vi "SQLiteConfig.vi"(4 "ConfigCommand":T2, 5 "error in (no error)":errorcluster, 7 "KeyDataIn":string, 8 "Parameter":T1) -> (0 "error out":errorcluster, 1 "All Data":string[][](array[string]), 2 "KeyData":string, 3 "AvailableVersions":string[](array[string]))   [LabVIEW 2023]
doc: "*-----------------------------------------------------\n* Author: SWatts\n*\n* VI Description: Configuration dialog\n* \n*\n* Error handling: All errors passed out\n*\n* Pre-condition: \n*\n* Post-condition: None\n*\n* Revision History:\n*\n* Rev Date Author Description \n* 01 30/04/2014 SWatts First issue\n*\n*-----------------------------------------------------"
uses:
  Datamanager.ctl
  Controls/SystemConfigData.ctl
  Database/SystemdBCommands.ctl
  System Config Data Manager Parameter.ctl
  ConfigCommand.ctl
panel:
  out "KeyNames":string[](array[string])
  # "Local"
  # "Output"
  # "Input"
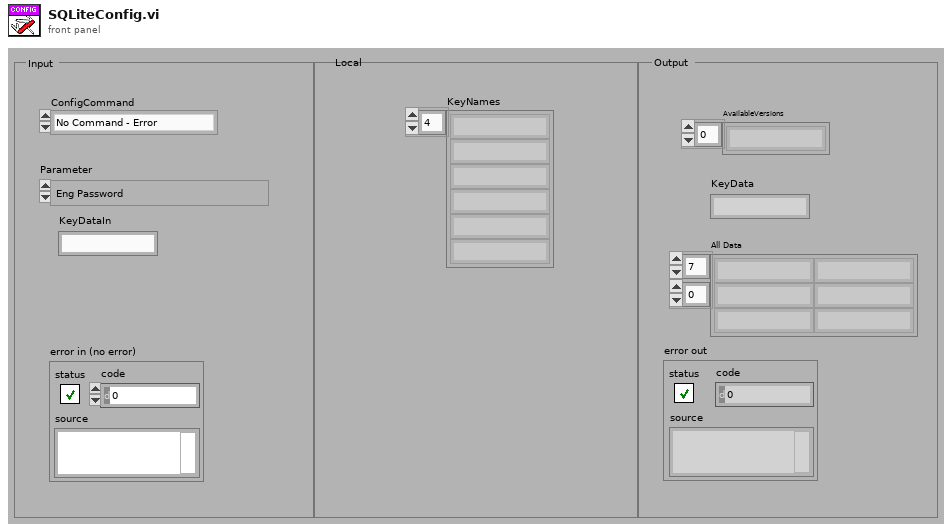
[diagram p1: front panel]
types:
  T1 = typedef "System Config Data Manager Parameter.ctl" = enum16{"Eng Password", "DSN Connection", "User Password", "RunStatus", "InitialDataPath", "helpFilePath", "ErrorFilepath", "DatalogPath", "Hello"}
  T2 = typedef "ConfigCommand.ctl" = enum16{"No Command - Error", "Initialise Config SQLite", "Save Config", "Get Key", "Set Key", "Update Key", "Get Latest Config Data", "Get Config Data for Version", "Get Default Config Data"}
  T3 = typedef "Datamanager.ctl" = enum16{"System Config"}
  T4 = typedef "SystemConfigData.ctl" = cluster{"KeyNames":string[], "Section":string, "Version":string, "KeyData":string[]}
  T5 = typedef "SystemdBCommands.ctl" = enum16{"No Command - Error", "Set Filepath", "Connect dB", "Disconnect dB", "Start Transaction", "Commit", "Rollback", "Describe Table", "Select All From Table", "Fetch Query", "Count Records In Table", "Get User Information", "Get System Config", "Insert New System Config", "UPDATE User Info", "Insert New User", "Get Versions", "Update Key", "Set Version to Default", "Get Default Version", "INSERT Error", "UPDATE Error", "DELETE Errors", "Get All Errors", "Get #Errors for Error"}
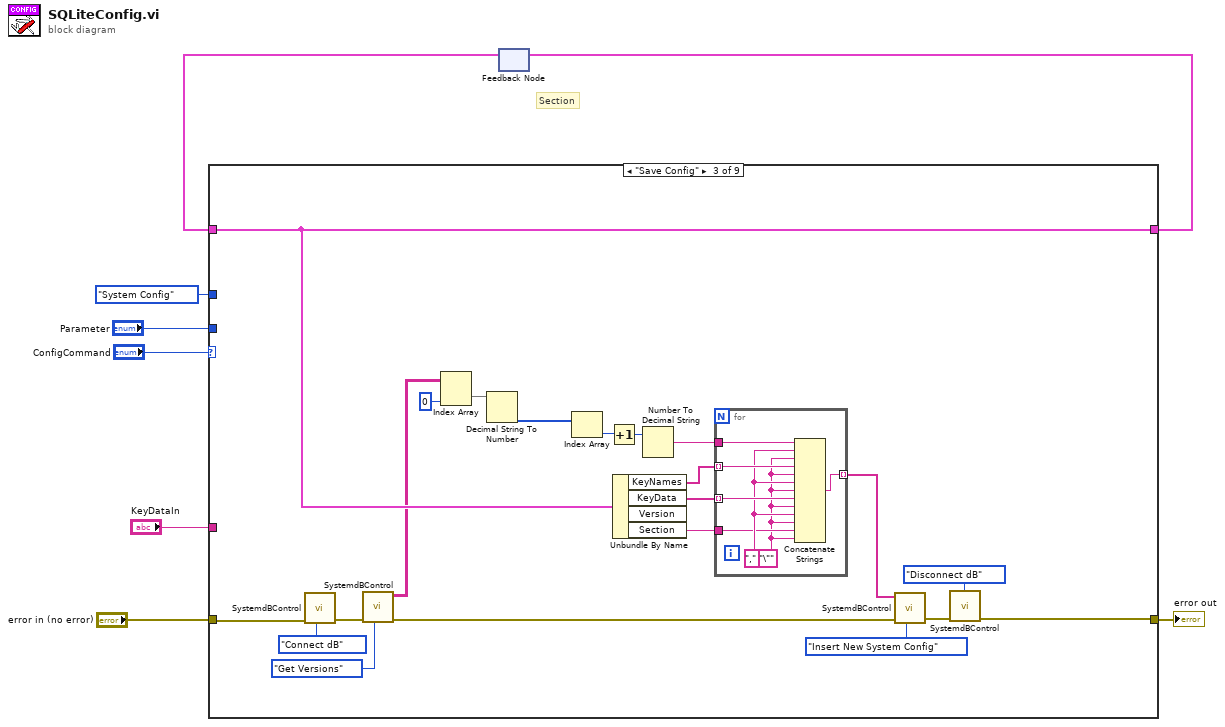
[diagram p0: block diagram]
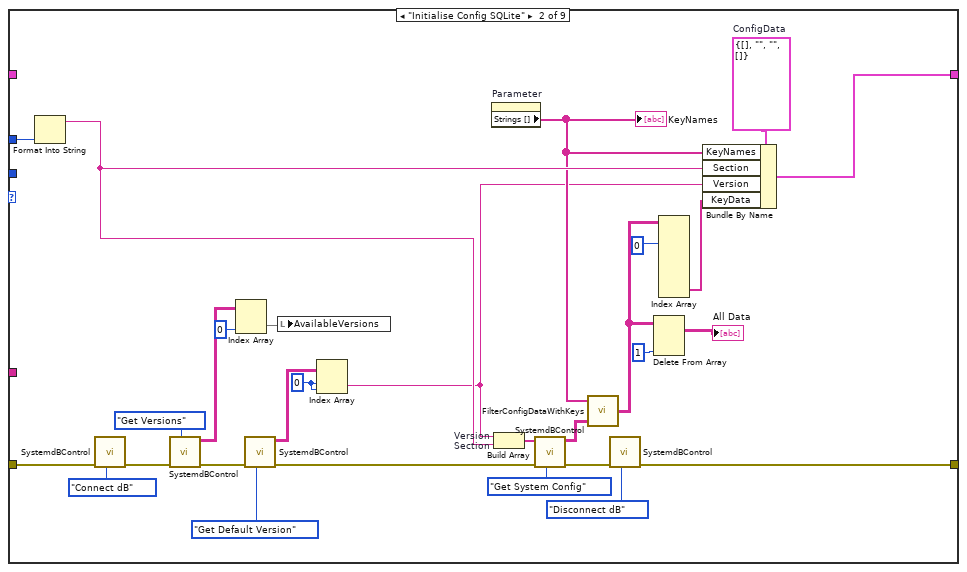
[diagram p3: hidden frame]
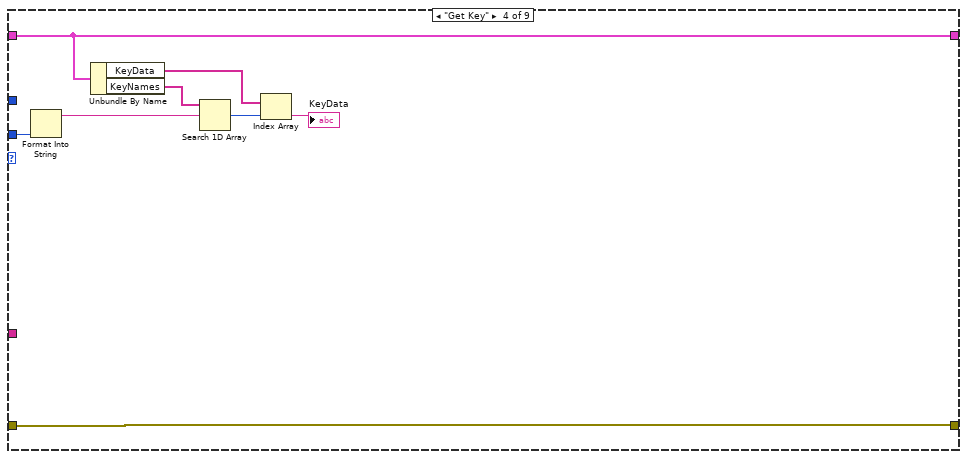
[diagram p4: hidden frame]
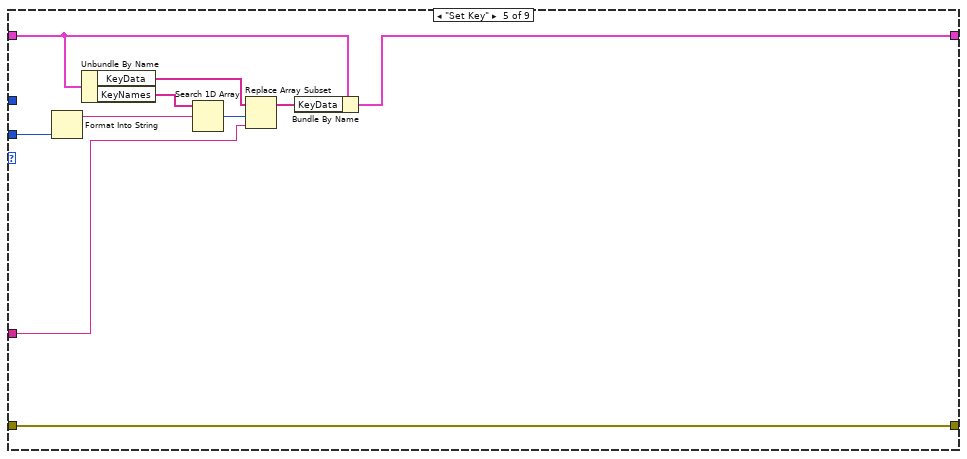
[diagram p5: hidden frame]
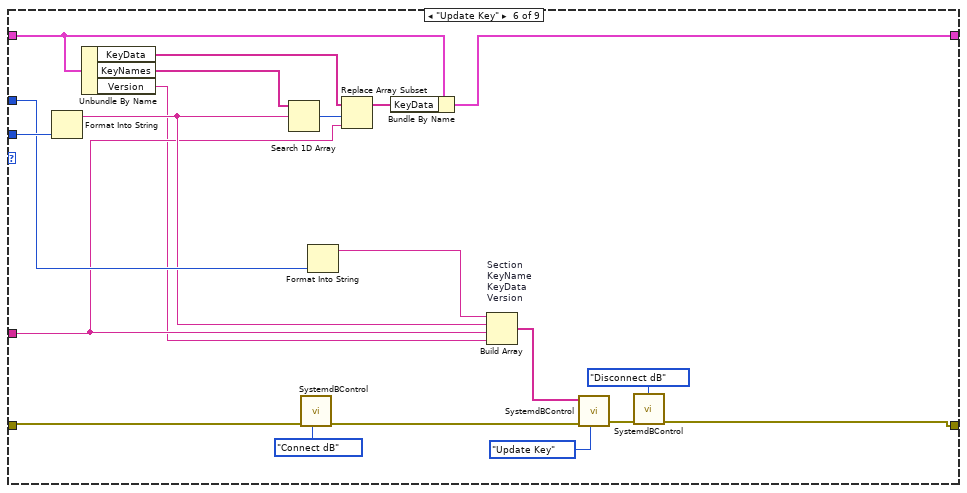
[diagram p6: hidden frame]
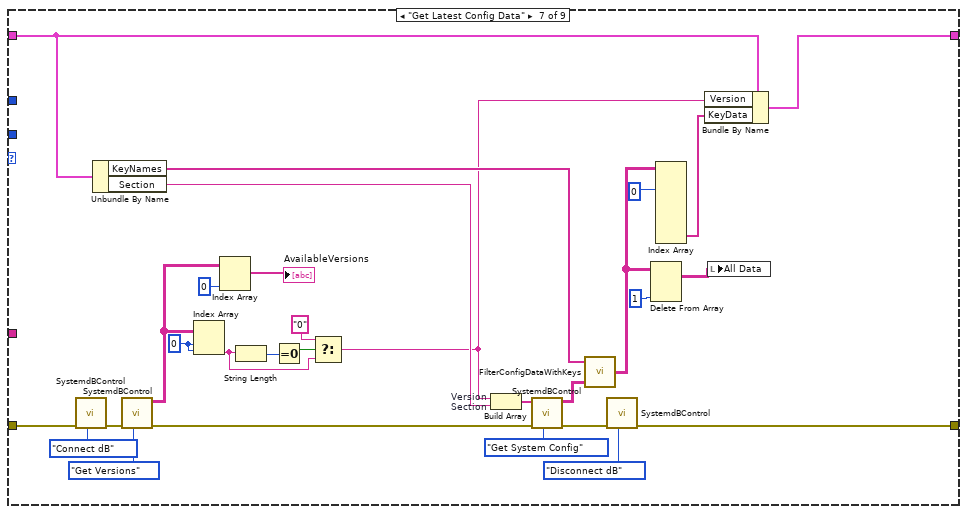
[diagram p7: hidden frame]
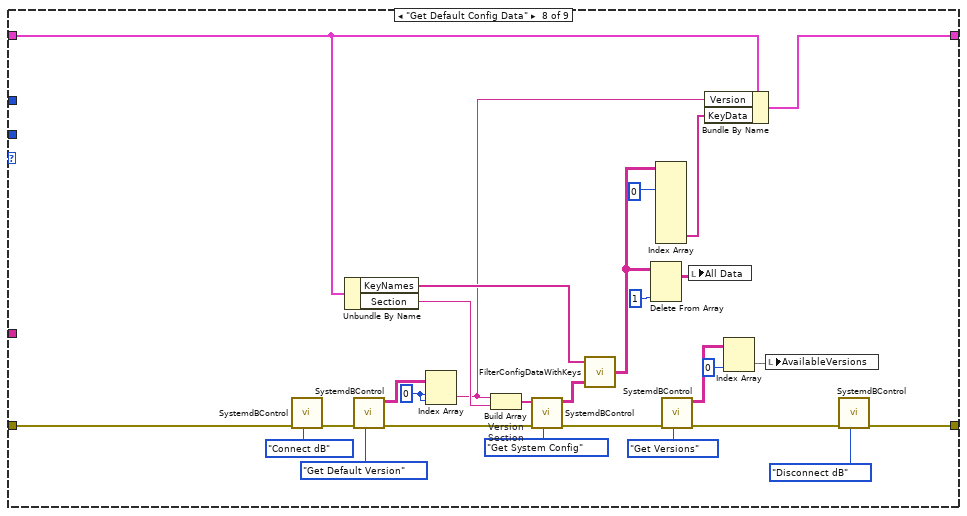
[diagram p8: hidden frame]
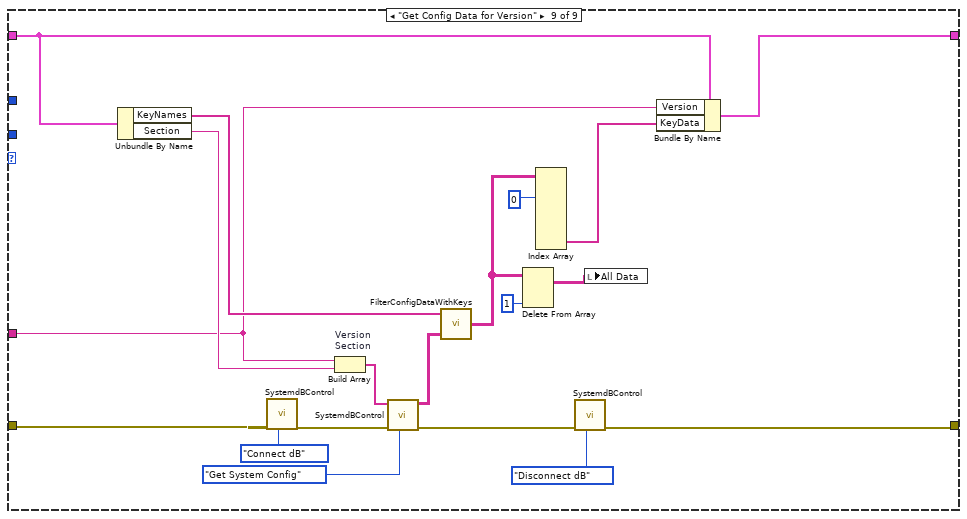
[diagram p9: hidden frame]
diagram:
  # "Section"
  n1 = feedback #1() -> (w1:T4)  [unwired: 1 in]
  n2 = case shown="\"Save Config\"" "ConfigCommand" {
    tunnel: "error in (no error)" -> [w10 w21 w50 w74 w84 w94 w111 w146 w168]
    tunnel: "Parameter" -> [_ _ _ w75 w85 w105 _ _ _]
    tunnel: [w10 w18 w49 w74 w84 w93 w107 w142 w167] -> w5
    tunnel: "KeyDataIn" -> [_ _ _ _ w78 w87 _ _ w164]
    tunnel: Datamanager."System Config" ("Section") -> [_ w39 _ _ _ w90 _ _ _]
    tunnel: [w9 w22 w48 w68 w77 w100 w109 w144 w165] -> w2
    tunnel: w1 -> [w9 _ w48 w68 w76 w99 w110 w145 w166]
    frame "No Command - Error", Default {
    }
    frame "Initialise Config SQLite" {
      w32 = 0 ("index (row)")
      w24 = T4 {"KeyNames"=[], "Section"="", "Version"="", "KeyData"=[]}  # ConfigData
      n3 = Format Into String(w39) -> (resulting string=w20:string)  [unwired: 3 in, 1 out]
      n4 = call "SystemdBControl.vi"("Command"=SystemdBCommands."Connect dB", "error in (no error)"=w21) -> ("error out"=w16:errorcluster)  [unwired: 5 in, 2 out]
      n5 = call "SystemdBControl.vi"("Command"=SystemdBCommands."Get Versions", "error in (no error)"=w16) -> ("error out"=w15:errorcluster, "Data Out"=w13:string[][])  [unwired: 5 in, 1 out]
      n6 = Index Array(array=w13, index (col)=0 ("disabled index (col)")) -> (element=w11:string[])  [unwired: 1 in]
      n7 = call "SystemdBControl.vi"("Command"=SystemdBCommands."Get Default Version", "error in (no error)"=w15) -> ("error out"=w30:errorcluster, "Data Out"=w33:string[][])  [unwired: 5 in, 1 out]
      n8 = local write "AvailableVersions"(w11) -> ()
      n9 = Index Array(array=w33, index (row)=w32, index (col)=w32) -> (element=w17:string)
      n10 = property on="Parameter" class="Enum (strict)"() -> ("Strings []"=w19:string[])  [unwired: 2 in, 2 out]
      "KeyNames" <- w19
      n11 = Build Array "Version\nSection"(w17, w20) -> (w35:string[])
      n12 = call "SystemdBControl.vi"("Command"=SystemdBCommands."Get System Config", "error in (no error)"=w30, "Data In"=w35) -> ("error out"=w28:errorcluster, "Data Out"=w34:string[][])  [unwired: 4 in, 1 out]
      n13 = call "FilterConfigDataWithKeys.vi"("Selected Items"=w34, "Keys"=w19) -> ("Filtered Selected Items"=w37:string[][])  [unwired: 3 in]
      n14 = call "SystemdBControl.vi"("Command"=SystemdBCommands."Disconnect dB", "error in (no error)"=w28) -> ("error out"=w18:errorcluster)  [unwired: 5 in, 2 out]
      n15 = Delete From Array(array=w37, index (col)=1 ("disabled index (col)")) -> (array with subset deleted=→"All Data":string[][])  [unwired: 2 in, 1 out]
      n16 = Index Array(array=w37, index (col) #1=0 ("index (row)")) -> (element #4=w38:string[])  [unwired: 7 in, 3 out]
      n17 = Bundle By Name(cluster=w24, "KeyNames"=w19, "Section"=w20, "Version"=w17, "KeyData"=w38) -> (w22:T4)
    }
    frame "Save Config" {
      n18 = call "SystemdBControl.vi"("Command"=SystemdBCommands."Connect dB", "error in (no error)"=w50) -> ("error out"=w47:errorcluster)  [unwired: 5 in, 2 out]
      n19 = call "SystemdBControl.vi"("Command"=SystemdBCommands."Get Versions", "error in (no error)"=w47) -> ("error out"=w42:errorcluster, "Data Out"=w44:string[][])  [unwired: 5 in, 1 out]
      n20 = Index Array(array=w44, index (col)=0 ("disabled index (col)")) -> (element=w43:string[])  [unwired: 1 in]
      n21 = Decimal String To Number(string=w43) -> (number=w40:i32[])  [unwired: 2 in, 1 out]
      n22 = Index Array(array=w40) -> (element=w41:i32)  [unwired: 1 in]
      n23 = Increment(x=w41) -> (x+1=w56:i32)
      n24 = Unbundle By Name(w48) -> ("KeyNames"=w59:string[], "KeyData"=w60:string[], "Section"=w58:string)  [unwired: 1 out]
      n25 = Number To Decimal String(number=w56) -> (decimal integer string=w52:string)  [unwired: 1 in]
      n26 = for {
        tunnel: w60 -> [w67] mode=indexing
        tunnel: [w66] -> w51 mode=indexing
        tunnel: w59 -> [w65] mode=indexing
        tunnel: w52 -> [w64]
        tunnel: w58 -> [w62]
        w63 = "," ("string")
        w61 = "\"" ("string")
        n27 = Concatenate Strings(w64, w63, w61, w65, w61, w63, w61, w67, w61, w63, w61, w62, w61) -> (w66:string)
      }
      n28 = call "SystemdBControl.vi"("Command"=SystemdBCommands."Insert New System Config", "error in (no error)"=w42, "Data In"=w51) -> ("error out"=w53:errorcluster)  [unwired: 4 in, 2 out]
      n29 = call "SystemdBControl.vi"("Command"=SystemdBCommands."Disconnect dB", "error in (no error)"=w53) -> ("error out"=w49:errorcluster)  [unwired: 5 in, 2 out]
    }
    frame "Get Key" {
      n30 = Format Into String(w75) -> (resulting string=w70:string)  [unwired: 3 in, 1 out]
      n31 = Unbundle By Name(w68) -> ("KeyData"=w73:string[], "KeyNames"=w72:string[])
      n32 = Search 1D Array(1D array=w72, element=w70) -> (index of element=w71:i32)  [unwired: 1 in]
      n33 = Index Array(array=w73, index=w71) -> (element=→"KeyData":string)
    }
    frame "Set Key" {
      n34 = Format Into String(w85) -> (resulting string=w79:string)  [unwired: 3 in, 1 out]
      n35 = Unbundle By Name(w76) -> ("KeyData"=w82:string[], "KeyNames"=w81:string[])
      n36 = Search 1D Array(1D array=w81, element=w79) -> (index of element=w80:i32)  [unwired: 1 in]
      n37 = Replace Array Subset(array=w82, new element=w78, index=w80) -> (w83:string[])
      n38 = Bundle By Name(cluster=w76, "KeyData"=w83) -> (w77:T4)
    }
    frame "Update Key" {
      n39 = Format Into String(w105) -> (resulting string=w88:string)  [unwired: 3 in, 1 out]
      n40 = Unbundle By Name(w99) -> ("KeyData"=w103:string[], "KeyNames"=w102:string[], "Version"=w86:string)
      n41 = Search 1D Array(1D array=w102, element=w88) -> (index of element=w101:i32)  [unwired: 1 in]
      n42 = call "SystemdBControl.vi"("Command"=SystemdBCommands."Connect dB", "error in (no error)"=w94) -> ("error out"=w97:errorcluster)  [unwired: 5 in, 2 out]
      n43 = Format Into String(w90) -> (resulting string=w89:string)  [unwired: 3 in, 1 out]
      n44 = Replace Array Subset(array=w103, new element=w87, index=w101) -> (w104:string[])
      n45 = Bundle By Name(cluster=w99, "KeyData"=w104) -> (w100:T4)
      n46 = Build Array "Section\nKeyName\nKeyData\nVersion"(w89, w88, w87, w86) -> (w91:string[])
      n47 = call "SystemdBControl.vi"("Command"=SystemdBCommands."Update Key", "error in (no error)"=w97, "Data In"=w91) -> ("error out"=w95:errorcluster)  [unwired: 4 in, 2 out]
      n48 = call "SystemdBControl.vi"("Command"=SystemdBCommands."Disconnect dB", "error in (no error)"=w95) -> ("error out"=w93:errorcluster)  [unwired: 5 in, 2 out]
    }
    frame "Get Latest Config Data" {
      w125 = 0 ("index (row)")
      n49 = call "SystemdBControl.vi"("Command"=SystemdBCommands."Connect dB", "error in (no error)"=w111) -> ("error out"=w123:errorcluster)  [unwired: 5 in, 2 out]
      n50 = Unbundle By Name(w110) -> ("KeyNames"=w132:string[], "Section"=w133:string)
      n51 = call "SystemdBControl.vi"("Command"=SystemdBCommands."Get Versions", "error in (no error)"=w123) -> ("error out"=w122:errorcluster, "Data Out"=w126:string[][])  [unwired: 5 in, 1 out]
      n52 = Index Array(array=w126, index (row)=w125, index (col)=w125) -> (element=w114:string)
      n53 = Index Array(array=w126, index (col)=0 ("disabled index (col)")) -> (element=→"AvailableVersions":string[])  [unwired: 1 in]
      n54 = String Length(string=w114) -> (length=w113:i32)
      n55 = Equal To 0?(x=w113) -> (x = 0?=w112:bool)
      n56 = Select(t="0" ("element"), s=w112, f=w114) -> (s? t:f=w115:string)
      n57 = Build Array "Version\nSection"(w115, w133) -> (w129:string[])
      n58 = call "SystemdBControl.vi"("Command"=SystemdBCommands."Get System Config", "error in (no error)"=w122, "Data In"=w129) -> ("error out"=w120:errorcluster, "Data Out"=w128:string[][])  [unwired: 4 in, 1 out]
      n59 = call "FilterConfigDataWithKeys.vi"("Selected Items"=w128, "Keys"=w132) -> ("Filtered Selected Items"=w131:string[][])  [unwired: 3 in]
      n60 = call "SystemdBControl.vi"("Command"=SystemdBCommands."Disconnect dB", "error in (no error)"=w120) -> ("error out"=w107:errorcluster)  [unwired: 5 in, 2 out]
      n61 = Delete From Array(array=w131, index (col)=1 ("disabled index (col)")) -> (array with subset deleted=w108:string[][])  [unwired: 2 in, 1 out]
      n62 = Index Array(array=w131, index (col) #1=0 ("index (row)")) -> (element #4=w134:string[])  [unwired: 7 in, 3 out]
      n63 = Bundle By Name(cluster=w110, "Version"=w115, "KeyData"=w134) -> (w109:T4)
      n64 = local write "All Data"(w108) -> ()
    }
    frame "Get Default Config Data" {
      w154 = 0 ("index (row)")
      n65 = call "SystemdBControl.vi"("Command"=SystemdBCommands."Connect dB", "error in (no error)"=w146) -> ("error out"=w152:errorcluster)  [unwired: 5 in, 2 out]
      n66 = Unbundle By Name(w145) -> ("KeyNames"=w160:string[], "Section"=w161:string)
      n67 = call "SystemdBControl.vi"("Command"=SystemdBCommands."Get Default Version", "error in (no error)"=w152) -> ("error out"=w151:errorcluster, "Data Out"=w155:string[][])  [unwired: 5 in, 1 out]
      n68 = Index Array(array=w155, index (row)=w154, index (col)=w154) -> (element=w141:string)
      n69 = Build Array "Version\nSection"(w141, w161) -> (w157:string[])
      n70 = call "SystemdBControl.vi"("Command"=SystemdBCommands."Get System Config", "error in (no error)"=w151, "Data In"=w157) -> ("error out"=w136:errorcluster, "Data Out"=w156:string[][])  [unwired: 4 in, 1 out]
      n71 = call "FilterConfigDataWithKeys.vi"("Selected Items"=w156, "Keys"=w160) -> ("Filtered Selected Items"=w159:string[][])  [unwired: 3 in]
      n72 = Delete From Array(array=w159, index (col)=1 ("disabled index (col)")) -> (array with subset deleted=w143:string[][])  [unwired: 2 in, 1 out]
      n73 = Index Array(array=w159, index (col) #1=0 ("index (row)")) -> (element #4=w162:string[])  [unwired: 7 in, 3 out]
      n74 = call "SystemdBControl.vi"("Command"=SystemdBCommands."Get Versions", "error in (no error)"=w136) -> ("error out"=w135:errorcluster, "Data Out"=w140:string[][])  [unwired: 5 in, 1 out]
      n75 = local write "All Data"(w143) -> ()
      n76 = Bundle By Name(cluster=w145, "Version"=w141, "KeyData"=w162) -> (w144:T4)
      n77 = Index Array(array=w140, index (col)=0 ("disabled index (col)")) -> (element=w138:string[])  [unwired: 1 in]
      n78 = local write "AvailableVersions"(w138) -> ()
      n79 = call "SystemdBControl.vi"("Command"=SystemdBCommands."Disconnect dB", "error in (no error)"=w135) -> ("error out"=w142:errorcluster)  [unwired: 5 in, 2 out]
    }
    frame "Get Config Data for Version" {
      n80 = Unbundle By Name(w166) -> ("KeyNames"=w178:string[], "Section"=w179:string)
      n81 = call "SystemdBControl.vi"("Command"=SystemdBCommands."Connect dB", "error in (no error)"=w168) -> ("error out"=w181:errorcluster)  [unwired: 5 in, 2 out]
      n82 = Build Array "Version\nSection"(w164, w179) -> (w175:string[])
      n83 = call "SystemdBControl.vi"("Command"=SystemdBCommands."Get System Config", "error in (no error)"=w181, "Data In"=w175) -> ("error out"=w172:errorcluster, "Data Out"=w174:string[][])  [unwired: 4 in, 1 out]
      n84 = call "FilterConfigDataWithKeys.vi"("Selected Items"=w174, "Keys"=w178) -> ("Filtered Selected Items"=w177:string[][])  [unwired: 3 in]
      n85 = Delete From Array(array=w177, index (col)=1 ("disabled index (col)")) -> (array with subset deleted=w163:string[][])  [unwired: 2 in, 1 out]
      n86 = Index Array(array=w177, index (col) #1=0 ("index (row)")) -> (element #4=w180:string[])  [unwired: 7 in, 3 out]
      n87 = call "SystemdBControl.vi"("Command"=SystemdBCommands."Disconnect dB", "error in (no error)"=w172) -> ("error out"=w167:errorcluster)  [unwired: 5 in, 2 out]
      n88 = local write "All Data"(w163) -> ()
      n89 = Bundle By Name(cluster=w166, "Version"=w164, "KeyData"=w180) -> (w165:T4)
    }
  }
  "error out" <- w5
  n90 = feedback-in #1(w2) -> ()
